vi "Handle TCP Message.vi"(7 "TCPMessageAPI":refnum<class "TCPMessageAPI.lvclass">, 8 "error in (no error)":errorcluster, 10 "TcpPayload":T1, 11 "Constellation Command Handler in":refnum<class "Constellation Command Handler.lvclass">) -> (0 "error out":errorcluster, 3 "Constellation Command Handler out":refnum<class "Constellation Command Handler.lvclass">)   [LabVIEW 2023, in "VectoScratch.lvlib" / "Constellation Command Handler.lvclass"]
uses:
  Vecto/TCPMessageService/TCPMessageAPI.lvclass
  Vecto/proto/TcpPayload/Data.ctl
  Constellation Command Handler.lvclass
  Constellation Command Handler.lvclass/Constellation Command Handler.ctl
  Vecto/proto/ConstellationCommand/ConstellationCommand.lvlib
  Vecto/proto/TcpPayload/TcpPayload.lvlib
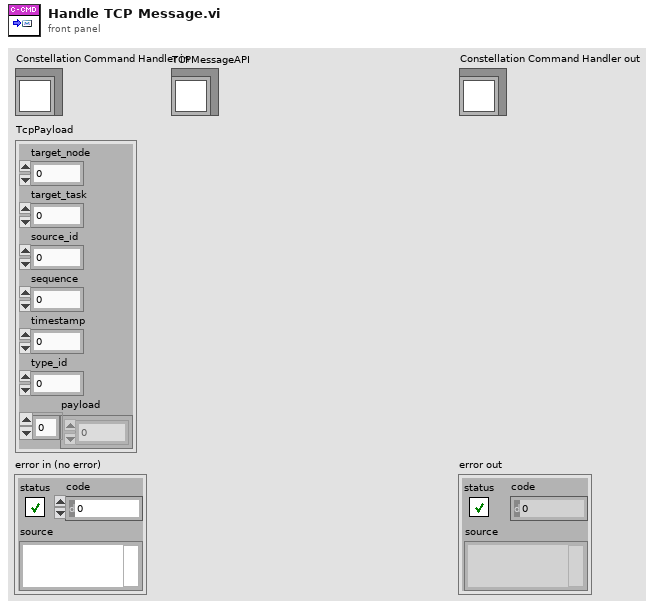
[diagram p1: front panel]
types:
  T1 = typedef "TcpPayload.lvlib/Data.ctl" = cluster{"target_node":u32, "target_task":u32, "source_id":u32, "sequence":u32, "timestamp":u64, "type_id":u32, "payload":u8[]}
  T2 = typedef "ConstellationCommand.lvlib/Data.ctl" = cluster{"Target Module":string, "Command":string, "Data":string[], "Time Stamp":timestamp}
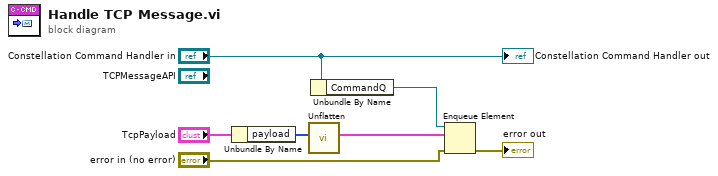
[diagram p0: block diagram]
diagram:
  n1 = Unbundle By Name("TcpPayload") -> ("payload"=w6:u8[])
  n2 = call "Unflatten.vi"("Buffer"=w6) -> ("Command Data"=w3:T2)  [unwired: 9 in, 1 out]
  n3 = Unbundle By Name("Constellation Command Handler in") -> ("CommandQ"=w4:refnum<queue>)
  n4 = Enqueue Element(queue=w4, element=w3, error in (no error)="error in (no error)") -> (error out=→"error out":errorcluster)  [unwired: 1 in, 2 out]
  "Constellation Command Handler out" <- "Constellation Command Handler in"
